vi "DriveSetGyroZero.vi"(8 "error in (no error)":errorcluster) -> (0 "error out":errorcluster)   [LabVIEW 2023]
doc: "Set GyroZero\n\nInputs:\n--GyroZero--Double--set gyro zero"
uses:
  DriveGlobal.vi
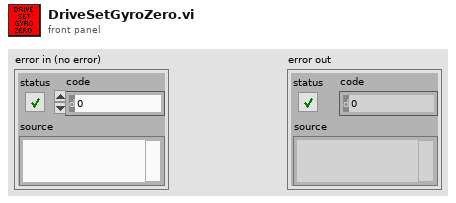
[diagram p1: front panel]
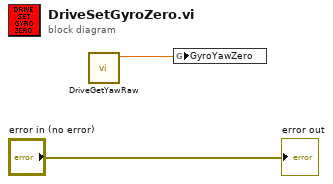
[diagram p0: block diagram]
diagram:
  n1 = call "DriveGetYawRaw.vi"() -> ("YawRaw"=w1:dbl)  [unwired: 11 in]
  n2 = global write "DriveGlobal.vi" "GyroYawZero"(w1) -> ()
  "error out" <- "error in (no error)"
